vi "svx_Colormap Draw Frequency.vi"(0 "color map ref in":refnum<vi>, 1 "Display Frequency":bool=TRUE, 3 "frequencytext":bool=TRUE, 5 "picture in":picture, 7 "speed profile":cluster{"time [s]":dbl[], "speed [rpm]":dbl[]} {"speed [rpm]" format="%.2f"; "time [s]" format="%.2f"}, 9 "Frequency Type":dbl[](array[numeric]), 11 "plot type":T3(ring), 12 "Line Configure":T2={"Line"={"Width"=1, "Style"=enum."Solid"}, "color"=0}, 14 "Text Configure":T1) -> (4 "color map ref out":refnum<vi>, 6 "picture out":picture)   [LabVIEW 2017, in "SVX Colormap.xctl"]
uses:
  <vilib>/addons/_XControls/Colormap/SVX Colormap.xctl
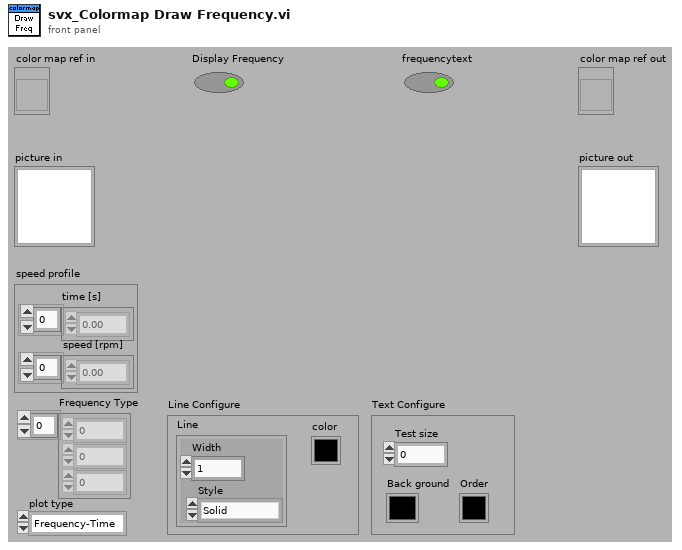
[diagram p1: front panel]
types:
  T1 = cluster{"Test size":i16, "Order":u32, "Back ground":u32}
  T2 = cluster{"Line":cluster{"Width":u16, "Style":enum32{"Solid", "Dash", "Dot", "DashDot", "DashDotDot"}}, "color":u32}
  T3 = enum16{"Frequency-Time", "Time-Frequency", "Order-Time", "Time-Order", "Frequency-RPM", "RPM-Frequency", "Order-RPM", "RPM-Order"}
  T4 = typedef "LVBoundsTypeDef.ctl" = cluster{"Width":u32, "Height":u32}
  T5 = cluster{"XScale.Minimum":dbl, "XScale.Maximum":dbl, "YScale.Minimum":dbl, "YScale.Maximum":dbl}
  T6 = cluster{"Width":u16, "Style":enum32{"Solid", "Dash", "Dot", "DashDot", "DashDotDot"}}
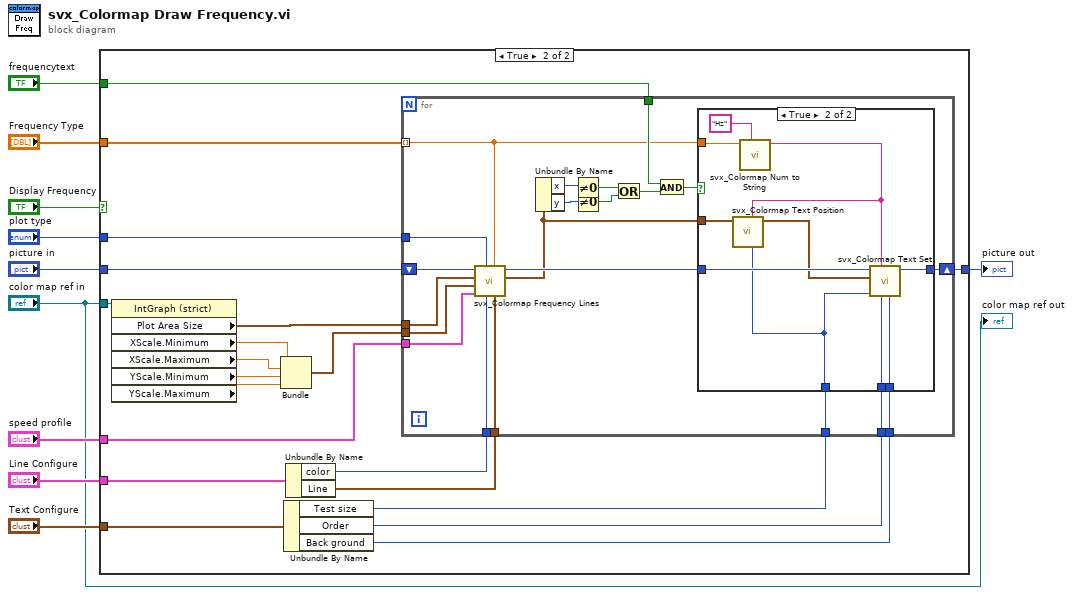
[diagram p0: block diagram]
diagram:
  n1 = case shown="True" "Display Frequency" {
    tunnel: [w11 w31] -> w8
    tunnel: "picture in" -> [w11 w30]
    tunnel: "plot type" -> [_ w29]
    tunnel: "frequencytext" -> [_ w28]
    tunnel: "Frequency Type" -> [_ w27]
    tunnel: "speed profile" -> [_ w26]
    tunnel: "Line Configure" -> [_ w25]
    tunnel: "Text Configure" -> [_ w22]
    tunnel: "color map ref in" -> [_ w14]
    frame False {
    }
    frame True {
      n2 = property class="IntGraph (strict)"(reference=w14) -> ("Plot Area Size"=w13:T4, "XScale.Minimum"=w15:dbl, "XScale.Maximum"=w16:dbl, "YScale.Minimum"=w17:dbl, "YScale.Maximum"=w18:dbl)  [unwired: 1 in, 2 out]
      n3 = Bundle("XScale.Minimum"=w15, "XScale.Maximum"=w16, "YScale.Minimum"=w17, "YScale.Maximum"=w18) -> (w12:T5)  [unwired: 1 in]
      n4 = Unbundle By Name(w22) -> ("Test size"=w21:i16, "Order"=w20:u32, "Back ground"=w19:u32)
      n5 = Unbundle By Name(w25) -> ("color"=w24:u32, "Line"=w23:T6)
      n6 = for {
        tunnel: w29 -> [w38]
        shift-right: [w52] -> w31
        shift-left: w30 -> [w41]
        tunnel: w27 -> [w37] mode=indexing
        tunnel: w12 -> [w32]
        tunnel: w28 -> [w49]
        tunnel: w13 -> [w40]
        tunnel: w20 -> [w46]
        tunnel: w19 -> [w45]
        tunnel: w21 -> [w44]
        tunnel: w23 -> [w34]
        tunnel: w24 -> [w33]
        tunnel: w26 -> [w39]
        n7 = call <vilib>:"svx_Colormap Frequency Lines.vi"("pen"=w34, "Frequency Type"=w37, "color(black)"=w33, "plot type"=w38, "speed profile"=w39, "Range"=w32, "Plot Area:Size"=w40, "picture in"=w41) -> ("Begin"=w35:cluster{"x":i16, "y":i16}, "picture Out"=w36:picture)  [unwired: 2 in]
        n8 = Unbundle By Name(w35) -> ("x"=w50:i16, "y"=w51:i16)
        n9 = Not Equal To 0?(x=w50) -> (x != 0?=w48:bool)
        n10 = Not Equal To 0?(x=w51) -> (x != 0?=w42:bool)
        n11 = Or(x=w48, y=w42) -> (x .or. y?=w43:bool)
        n12 = And(x=w49, y=w43) -> (x .and. y?=w47:bool)
        n13 = case shown="True" w47 {
          tunnel: w36 -> [w53 w60]
          tunnel: [w53 w61] -> w52
          tunnel: w35 -> [_ w59]
          tunnel: w37 -> [_ w56]
          tunnel: w46 -> [_ w63]
          tunnel: w45 -> [_ w62]
          tunnel: w44 -> [_ w57]
          frame False {
          }
          frame True {
            n14 = call <vilib>:"svx_Colormap Num to String.vi"("Unit"="Hz", "Order"=w56) -> ("String"=w55:string)  [unwired: 8 in, 1 out]
            n15 = call <vilib>:"svx_Colormap Text Position.vi"("Test size"=w57, "String"=w55, "End"=w59) -> ("text position"=w58:cluster{"x":i16, "y":i16})  [unwired: 8 in]
            n16 = call <vilib>:"svx_Colormap Text Set.vi"("BG color(transparent)"=w62, "text color(black)"=w63, "text"=w55, "Size"=w57, "origin"=w58, "picture"=w60) -> ("new picture"=w61:picture)  [unwired: 5 in]
          }
        }
      }
    }
  }
  "picture out" <- w8
  "color map ref out" <- "color map ref in"
